vi "Time FGV.vi"(8 "error in (no error)":errorcluster, 9 "Enum":enum16{"initalise", "read", "write"}(ring), 10 "Countdown (s) in":dbl) -> (0 "error out":errorcluster, 2 "Countdown (s) out":dbl)   [LabVIEW 2020, in "Wait.lvlib"]
uses:
  Wait.lvlib
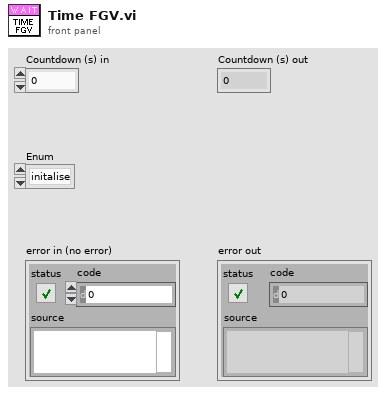
[diagram p1: front panel]
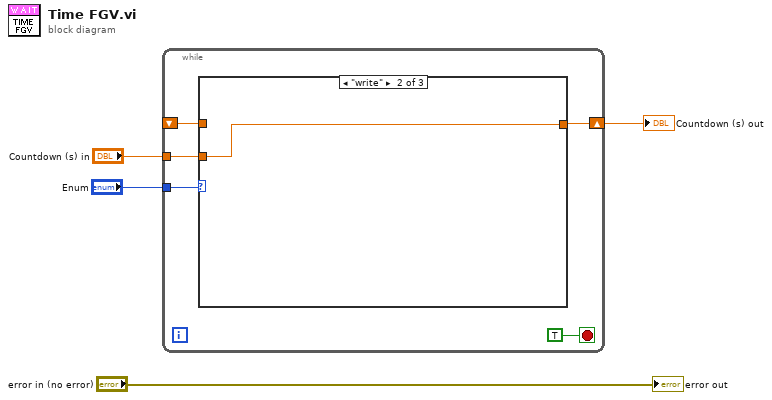
[diagram p0: block diagram]
diagram:
  n1 = while {
    tunnel: "Enum" -> [w9]
    tunnel: "Countdown (s) in" -> [w8]
    shift-right: [w5] -> w1
    shift-left: _ -> [w7]
    stop <- TRUE stop-if-true
    n2 = case shown="\"write\"" w9 {
      tunnel: w8 -> [_ w10 _]
      tunnel: w7 -> [_ _ w11]
      tunnel: [_ w10 w11] -> w5
      frame "initalise", Default {
      }
      frame "write" {
      }
      frame "read" {
      }
    }
  }
  "Countdown (s) out" <- w1
  "error out" <- "error in (no error)"
